vi "FF_AnkleTrajAdv.vi"(6 "Init":bool, 7 "dt":dbl=0.01 format="%0.2f", 8 "error in (no error)":errorcluster, 9 "AnkleVelocity":dbl[](array[numeric]), 10 "AnkleInGCS":dbl[](array[numeric]), 11 "Force Field Controller in":refnum<class "ForceField.lvclass">) -> (0 "error out":errorcluster, 1 "ClosestPoint":dbl[](array[numeric]), 2 "ForceXYZ":dbl[](array[numeric]), 3 "Force Field Controller out":refnum<class "ForceField.lvclass">, 4 "UpdateTrajPrev":bool, 5 "ForceNTD":dbl[](array[numeric]))   [LabVIEW 2015, in "ForceField.lvclass"]
uses:
  ForceField.lvclass
  ForceField.lvclass/ForceField.ctl
  TypeDef/TND.ctl
  <vilib>/ptbypt/NI_PtbyPt.lvlib
panel:
  in  "3D":bool
  in  "Adv?":bool=TRUE
  out "weightPrev":dbl
  out "ClosePt 2":dbl[](array[numeric])
  in  "HalfWindow 2":i32=35
  in  "dXmin":dbl=0.2 format="%#_13g"
  in  "HalfWindow 1":i32=35
  out "ClosePt 1":dbl[](array[numeric])
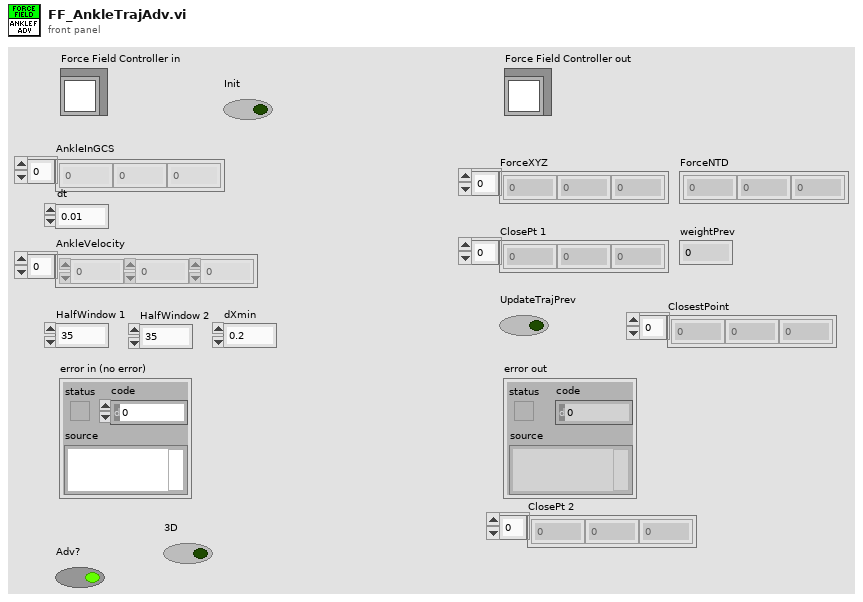
[diagram p1: front panel]
types:
  T1 = typedef "ForceField.lvclass/TND.ctl" = cluster{"Vt":dbl[], "Vn":dbl[], "Dmin":dbl}
  T2 = typedef "ForceField.lvclass/AnkleTrajPt.ctl" = cluster{"P1":dbl[], "P2":dbl[], "P1-P2":dbl[], "(P1-P2)^2":dbl}
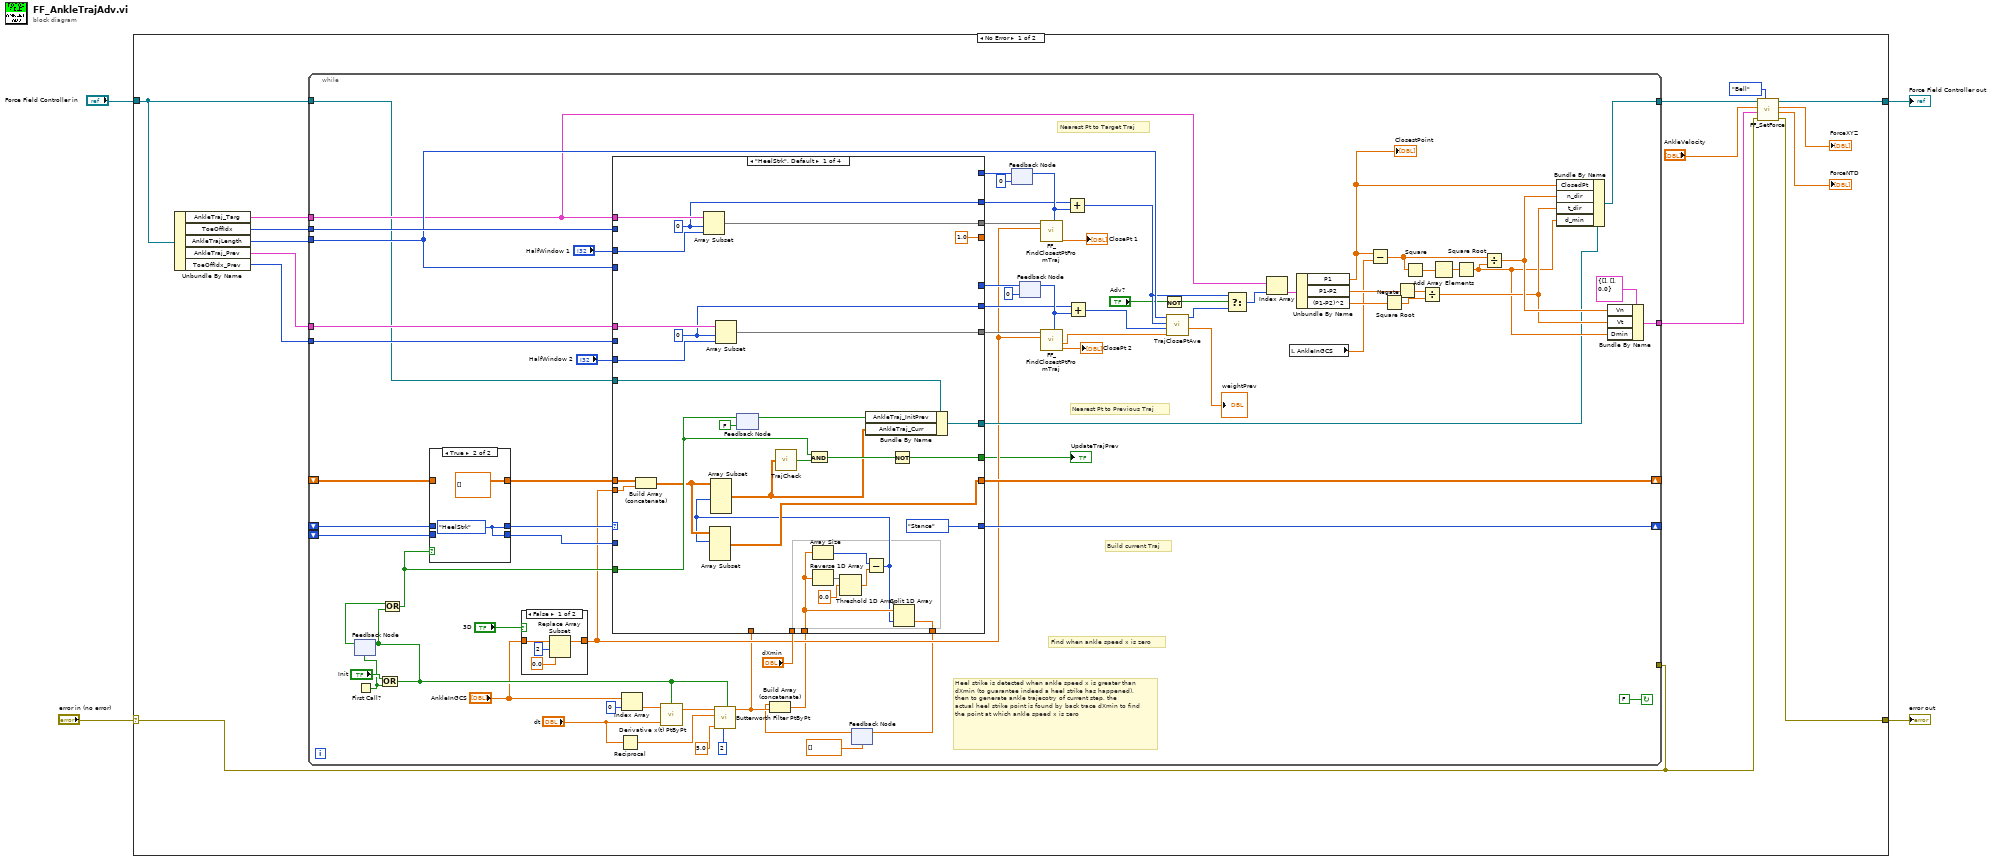
[diagram p0: block diagram]
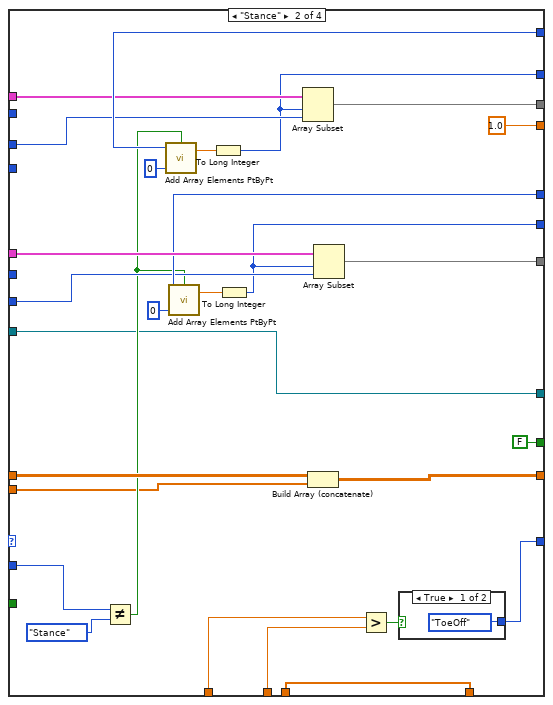
[diagram p3: hidden frame]
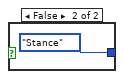
[diagram p4: hidden frame]
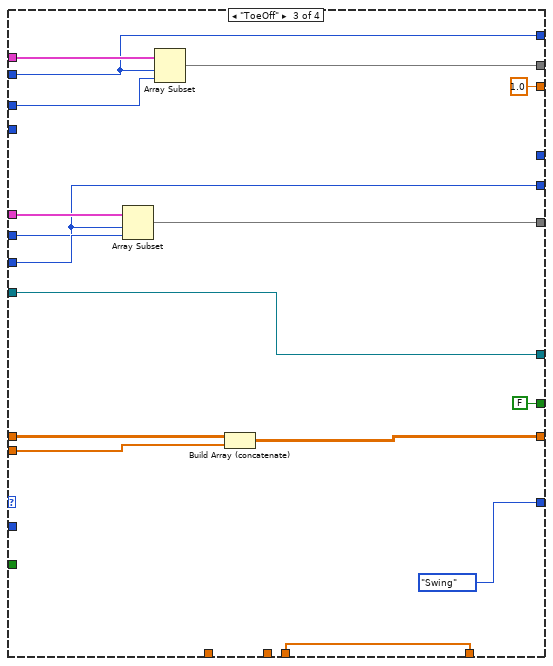
[diagram p5: hidden frame]
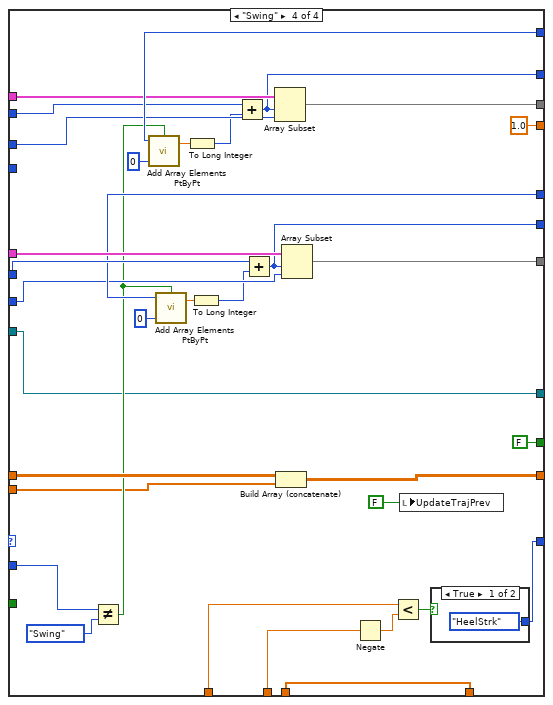
[diagram p6: hidden frame]
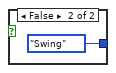
[diagram p7: hidden frame]
diagram:
  n1 = case shown="No Error" "error in (no error)" {
    selector: "error in (no error)" -> [w5 w219]
    tunnel: [w17 w219] -> w3
    tunnel: [w18 w218] -> w1
    tunnel: "Force Field Controller in" -> [w19 w218]
    frame No Error {
      n2 = Unbundle By Name(w19) -> ("AnkleTraj_Targ"=w15:T2[], "ToeOffIdx"=w14:i32, "AnkleTrajLength"=w13:i32, "AnkleTraj_Prev"=w7:T2[], "ToeOffIdx_Prev"=w6:i32)
      n3 = while {
        tunnel: w15 -> [w75]
        tunnel: w14 -> [w86]
        tunnel: w19 -> [w38]
        tunnel: [w95] -> w16
        shift-right: [w89] -> _
        shift-left: _ -> [w81]
        shift-left: _ -> [w79]
        shift-right: [w88] -> _
        shift-left: _ -> [w83]
        tunnel: w13 -> [w84]
        tunnel: w7 -> [w87]
        tunnel: w6 -> [w85]
        tunnel: [w62] -> w12
        tunnel: w5 -> [_]
        stop <- FALSE continue-if-true
        # "Heel strike is detected when ankle speed x is greater than dXmin (to guarantee indeed a heel strike has happened), then to generate ankle trajecotry of current step, the  actual heel strike point is found by back trace dXmin to find the point at which ankle speed x is zero"
        # "Find when ankle speed x is zero"
        # "Nearest Pt to Previous Traj"
        # "Build current Traj"
        # "Nearest Pt to Target Traj"
        n4 = First Call?() -> (First Call?: T/F=w76:bool)
        n5 = feedback #1(w76) -> (w77:bool)
        n6 = Or(x="Init", y=w76) -> (x .or. y?=w33:bool)
        n7 = feedback-in #1(w33) -> ()
        n8 = Or(x=w77, y=w33) -> (x .or. y?=w61:bool)
        n9 = case shown="True" w61 {
          tunnel: w83 -> [w215 _]
          tunnel: [w215 dbl[][] []] -> w82
          tunnel: w81 -> [w214 _]
          tunnel: [w214 w216] -> w80
          tunnel: w79 -> [w213 _]
          tunnel: [w213 w216] -> w78
          frame False {
          }
          frame True {
            w216 = enum16{"HeelStrk", "Stance", "ToeOff", "Swing"}."HeelStrk"
          }
        }
        n10 = case shown="False" "3D" {
          tunnel: "AnkleInGCS" -> [w99 w100]
          tunnel: [w98 w100] -> w27
          frame False {
            n11 = Replace Array Subset(array=w99, new element=0.0 ("new element/subarray"), index=2) -> (w98:dbl[])
          }
          frame True {
          }
        }
        n12 = Reciprocal(x="dt") -> (1/x=w31:dbl)
        n13 = Index Array(array="AnkleInGCS", index=0) -> (element=w92:dbl)
        n14 = call <vilib>:"Derivative x(t) PtByPt.vi"("initialize"=w33, "dt"="dt", "x"=w92) -> ("dx/dt"=w35:dbl)  [unwired: 1 in, 1 out]
        n15 = call <vilib>:"Butterworth Filter PtByPt.vi"("initialize"=w33, "order"=2, "low cutoff freq: fl"=5.0, "sampling freq: fs"=w31, "x"=w35) -> ("Filtered x"=w24:dbl)  [unwired: 4 in, 1 out]
        n16 = feedback #2(dbl[] []) -> (w23:dbl[])
        n17 = Build Array (concatenate)(w23, w24) -> (w20:dbl[])
        n18 = feedback #3(0 ("IndexOfClosePt")) -> (w59:i32)
        n19 = feedback #4(0 ("IndexOfClosePt")) -> (w53:i32)
        n20 = case shown="\"HeelStrk\", Default" w80 {
          tunnel: w75 -> [w127 w150 w170 w196]
          tunnel: "HalfWindow 1" -> [w128 w157 w174 w209]
          tunnel: [w130 w154 w176 w206] -> w57
          tunnel: [enum16{"HeelStrk", "Stance", "ToeOff", "Swing"}."Stance" w153 enum16{"HeelStrk", "Stance", "ToeOff", "Swing"}."Swing" w204] -> w89
          tunnel: w59 -> [_ w158 _ w210]
          tunnel: w24 -> [_ w152 _ w203]
          tunnel: w78 -> [_ w149 _ w202]
          tunnel: [1.0 1.0 1.0 1.0] -> _
          tunnel: "dXmin" -> [_ w147 _ w199]
          tunnel: w27 -> [w116 w133 w163 w179]
          tunnel: [w102 w146 w171 w197] -> w88
          tunnel: w82 -> [w105 w145 w172 w198]
          tunnel: w84 -> [_ _ _ _]
          tunnel: w87 -> [w125 w143 w169 w191]
          tunnel: "HalfWindow 2" -> [w124 w140 w167 w188]
          tunnel: [w123 w141 w168 w187] -> w52
          tunnel: w86 -> [_ _ w166 w194]
          tunnel: w53 -> [_ w142 _ w189]
          tunnel: w85 -> [_ _ w165 w190]
          tunnel: [w121 w135 w165 w185] -> w49
          tunnel: [w122 w136 w166 w184] -> w47
          tunnel: w61 -> [w112 _ _ _]
          tunnel: w38 -> [w119 w134 w164 w180]
          tunnel: [w117 w134 w164 w180] -> w37
          tunnel: [w114 FALSE FALSE FALSE] -> w25
          tunnel: [w106 w131 w161 w177] -> w21
          tunnel: w20 -> [w107 w131 w161 w177]
          frame "HeelStrk", Default {
            w121 = 0 ("index")
            w122 = 0 ("index")
            n21 = Build Array (concatenate)(w105, w116) -> (w103:dbl[][])
            n22 = Array Subset(array=w127, index=w122, length=w128) -> (w130:T2[])
            n23 = Array Subset(array=w125, index=w121, length=w124) -> (w123:T2[])
            n24 = feedback-in #5(w112) -> ()
            n25 = feedback #5(FALSE) -> (w118:bool)
            n26 = Array Size(array=w107) -> (size(s)=w109:i32)
            n27 = Reverse 1D Array(array=w107) -> (reversed array=w111:dbl[])
            n28 = Threshold 1D Array(2:0.0 ("threshold y"), 3:w111) -> (0:w108:dbl)  [unwired: 1 in]
            n29 = Subtract(x=w109, y=w108) -> (x-y=w101:i32)
            n30 = Array Subset(array=w103, index (row)=w101) -> (w102:dbl[][])  [unwired: 3 in]
            n31 = Array Subset(array=w103, length (row)=w101) -> (w104:dbl[][])  [unwired: 3 in]
            n32 = call "TrajCheck.vi"("TrajIn"=w104) -> ("GoodTrajectory?"=w113:bool)
            n33 = And(x=w112, y=w113) -> (x .and. y?=w115:bool)
            n34 = Bundle By Name(cluster=w119, "AnkleTraj_InitPrev"=w118, "AnkleTraj_Curr"=w104) -> (w117:refnum<class "ForceField.lvclass">)
            n35 = Not(x=w115) -> (.not. x?=w114:bool)
            n36 = Split 1D Array(array=w107, index=w101) -> (second subarray=w106:dbl[])  [unwired: 1 out]
          }
          frame "Stance" {
            n37 = Not Equal?(x=w149, y=enum16{"HeelStrk", "Stance", "ToeOff", "Swing"}."Stance") -> (x != y?=w139:bool)
            n38 = call <vilib>:"Add Array Elements PtByPt.vi"("initialize"=w139, "sample length"=0, "input data point"=w158) -> ("sum"=w138:dbl)  [unwired: 1 in, 1 out]
            n39 = call <vilib>:"Add Array Elements PtByPt.vi"("initialize"=w139, "sample length"=0, "input data point"=w142) -> ("sum"=w137:dbl)  [unwired: 1 in, 1 out]
            n40 = To Long Integer(number=w138) -> (32bit integer=w136:i32)
            n41 = To Long Integer(number=w137) -> (32bit integer=w135:i32)
            n42 = Array Subset(array=w150, index=w136, length=w157) -> (w154:T2[])
            n43 = Build Array (concatenate)(w145, w133) -> (w146:dbl[][])
            n44 = Array Subset(array=w143, index=w135, length=w140) -> (w141:T2[])
            n45 = Greater?(x=w152, y=w147) -> (0:w151:bool)
            n46 = case shown="True" w151 {
              tunnel: [enum16{"HeelStrk", "Stance", "ToeOff", "Swing"}."ToeOff" enum16{"HeelStrk", "Stance", "ToeOff", "Swing"}."Stance"] -> w153
              frame True {
              }
              frame False {
              }
            }
          }
          frame "ToeOff" {
            n47 = Array Subset(array=w169, index=w165, length=w167) -> (w168:T2[])
            n48 = Array Subset(array=w170, index=w166, length=w174) -> (w176:T2[])
            n49 = Build Array (concatenate)(w172, w163) -> (w171:dbl[][])
          }
          frame "Swing" {
            n50 = Not Equal?(x=w202, y=enum16{"HeelStrk", "Stance", "ToeOff", "Swing"}."Swing") -> (x != y?=w186:bool)
            n51 = call <vilib>:"Add Array Elements PtByPt.vi"("initialize"=w186, "sample length"=0, "input data point"=w210) -> ("sum"=w195:dbl)  [unwired: 1 in, 1 out]
            n52 = call <vilib>:"Add Array Elements PtByPt.vi"("initialize"=w186, "sample length"=0, "input data point"=w189) -> ("sum"=w193:dbl)  [unwired: 1 in, 1 out]
            n53 = To Long Integer(number=w195) -> (32bit integer=w183:i32)
            n54 = To Long Integer(number=w193) -> (32bit integer=w182:i32)
            n55 = Add(x=w194, y=w183) -> (x+y=w184:i32)
            n56 = Add(x=w190, y=w182) -> (x+y=w185:i32)
            n57 = Array Subset(array=w196, index=w184, length=w209) -> (w206:T2[])
            n58 = Build Array (concatenate)(w198, w179) -> (w197:dbl[][])
            n59 = Array Subset(array=w191, index=w185, length=w188) -> (w187:T2[])
            n60 = Negate(x=w199) -> (-x=w200:dbl)
            n61 = Less?(x=w203, y=w200) -> (x < y?=w205:bool)
            n62 = local write "UpdateTrajPrev"(FALSE ("UpdateTrajPrev")) -> ()
            n63 = case shown="True" w205 {
              tunnel: [enum16{"HeelStrk", "Stance", "ToeOff", "Swing"}."HeelStrk" enum16{"HeelStrk", "Stance", "ToeOff", "Swing"}."Swing"] -> w204
              frame True {
              }
              frame False {
              }
            }
          }
        }
        "UpdateTrajPrev" <- w25
        n64 = feedback-in #2(w21) -> ()
        n65 = call "FF_FindClosestPtFromTraj.vi"("AnkleInGCS"=w27, "AnkleTraj"=w57) -> ("ClosestPt"=→"ClosePt 1":dbl[], "IndexOfClosePt"=w48:i32)  [unwired: 5 in, 3 out]
        n66 = feedback-in #3(w48) -> ()
        n67 = call "FF_FindClosestPtFromTraj.vi"("AnkleInGCS"=w27, "AnkleTraj"=w52) -> ("ClosestPt"=→"ClosePt 2":dbl[], "DistanceToClosestPt"=w45:dbl, "IndexOfClosePt"=w50:i32)  [unwired: 5 in, 2 out]
        n68 = feedback-in #4(w50) -> ()
        n69 = Add(x=w47, y=w48) -> (x+y=w42:i32)
        n70 = Add(x=w49, y=w50) -> (x+y=w46:i32)
        n71 = Not(x="Adv?") -> (.not. x?=w40:bool)
        n72 = call "TrajClosePtAve.vi"("Dmin_Prev"=w45, "ClosePtIdx_Prev"=w46, "ClosePtIdx_Target"=w42, "TrajLength"=w84) -> ("weightPrev"=→"weightPrev":dbl, "ClosePtIdx_Ave"=w43:i32)  [unwired: 6 in]
        n73 = Select(t=w42, s=w40, f=w43) -> (s? t:f=w60:i32)
        n74 = Index Array(array=w75, index=w60) -> (element=w74:T2)
        n75 = local read "AnkleInGCS"() -> (w26:dbl[])
        n76 = Unbundle By Name(w74) -> ("P1"=w36:dbl[], "P1-P2"=w71:dbl[], "(P1-P2)^2"=w70:dbl)
        "ClosestPoint" <- w36
        n77 = Subtract(x=w36, y=w26) -> (x-y=w67:dbl[])
        n78 = Square Root(x=w70) -> (sqrt(x)=w72:dbl)
        n79 = Negate(x=w71) -> (-x=w73:dbl[])
        n80 = Square(x=w67) -> (x^2=w69:dbl[])
        n81 = Divide(x=w73, y=w72) -> (x/y=w64:dbl[])
        n82 = Add Array Elements(numeric array=w69) -> (sum=w68:dbl)
        n83 = Square Root(x=w68) -> (sqrt(x)=w63:dbl)
        n84 = Divide(x=w67, y=w63) -> (x/y=w65:dbl[])
        n85 = Bundle By Name(cluster=w37, "ClosedPt"=w36, "n_dir"=w65, "t_dir"=w64, "d_min"=w63) -> (w95:refnum<class "ForceField.lvclass">)
        n86 = Bundle By Name(cluster=T1 {"Vt"=[], "Vn"=[], "Dmin"=0.0} ("TND"), "Vn"=w65, "Vt"=w64, "Dmin"=w63) -> (w62:T1)
      }
      n87 = call "FF_SetForce.vi"("Enum"=enum16{"Linear", "Bell"}."Bell", "error in (no error)"=w5, "TND"=w12, "AnkleVelocity"="AnkleVelocity", "Force Field Controller in"=w16) -> ("error out"=w17:errorcluster, "ForceNTD"=→"ForceNTD":dbl[], "ForceXYZ"=→"ForceXYZ":dbl[], "Force Field Controller out"=w18:refnum<class "ForceField.lvclass">)  [unwired: 3 in]
    }
    frame Error {
    }
  }
  "error out" <- w3
  "Force Field Controller out" <- w1
